vi "RT_I2C Read.vi"(7 "Command":enum16{"Write", "Read", "Write&Read"}(ring)=enum."Read", 8 "error in":errorcluster, 9 "Number of Bytes to Read":u16, 10 "Input Array":u8[](array[numeric]), 11 "FPGA VI Reference In":T1) -> (0 "error out":errorcluster, 2 "Data":u8[](array[numeric]), 3 "FPGA VI Reference Out":T1)   [LabVIEW 2018]
uses:
  Data Def/RT_FPGA VI Reference.ctl
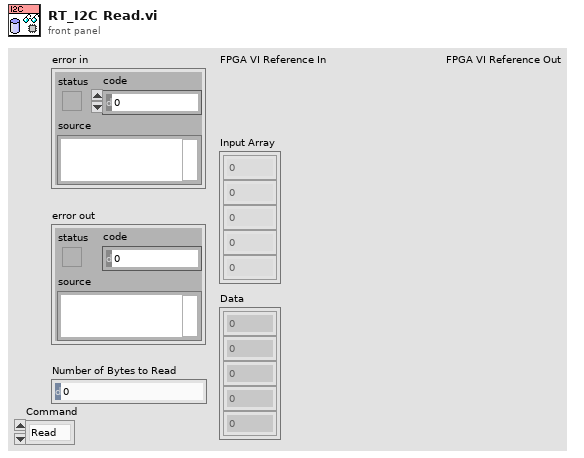
[diagram p1: front panel]
types:
  T1 = typedef "RT_FPGA VI Reference.ctl" = refnum<k20>
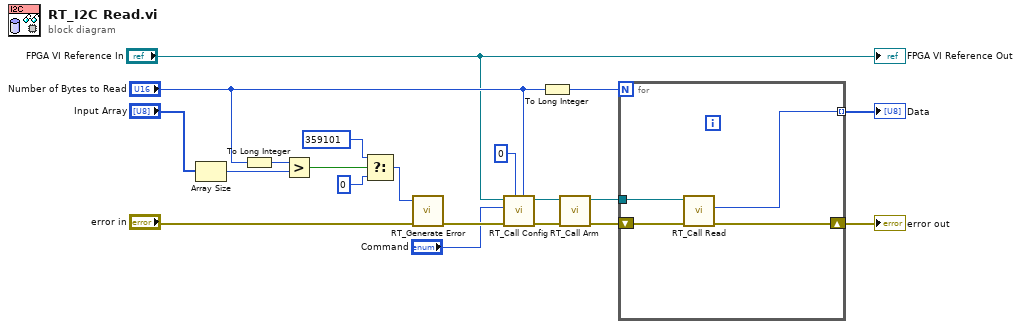
[diagram p0: block diagram]
diagram:
  n1 = Array Size(array="Input Array") -> (size(s)=w17:i32)
  n2 = To Long Integer(number="Number of Bytes to Read") -> (32bit integer=w9:i32)
  n3 = Greater?(x=w9, y=w17) -> (0:w16:bool)
  n4 = Select(t=359101, s=w16, f=0) -> (s? t:f=w10:i32)
  n5 = call "RT_Generate Error.vi"("error in (no error)"="error in", "Code"=w10) -> ("error out"=w13:errorcluster)  [unwired: 9 in]
  n6 = call "RT_Call Config.vi"("Number of Bytes to Read"="Number of Bytes to Read", "Number of Bytes to Write"=u16 0, "error in"=w13, "Command"="Command", "FPGA VI Reference In"="FPGA VI Reference In") -> ("error out"=w4:errorcluster, "FPGA VI Reference Out"=w5:T1)  [unwired: 5 in]
  n7 = To Long Integer(number="Number of Bytes to Read") -> (32bit integer=w7:i32)
  n8 = call "RT_Call Arm.vi"("error in"=w4, "FPGA VI Reference In"=w5) -> ("error out"=w3:errorcluster, "FPGA VI Reference Out"=w2:T1)  [unwired: 8 in]
  n9 = for {
    N: w7 -> [_]
    shift-right: [w23] -> w19
    shift-left: w3 -> [w24]
    tunnel: w2 -> [w22]
    tunnel: [w21] -> w1 mode=indexing
    n10 = call "RT_Call Read.vi"("error in"=w24, "FPGA VI Reference In"=w22) -> ("error out"=w23:errorcluster, "Data Out"=w21:u8)  [unwired: 7 in, 1 out]
  }
  "error out" <- w19
  "Data" <- w1
  "FPGA VI Reference Out" <- "FPGA VI Reference In"
